vi "fgv - fast counter.vi"(8 "error in (no error)":errorcluster, 10 "Write Data (0)":u16, 11 "Operation":enum16{"Read", "Write"}(ring)) -> (0 "error out":errorcluster, 2 "Read Data":u16)   [LabVIEW 2016]
panel:
  # "fgv - fast counter"
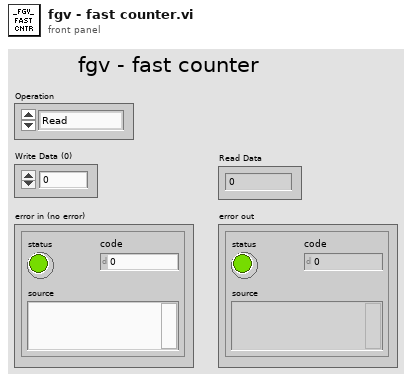
[diagram p1: front panel]
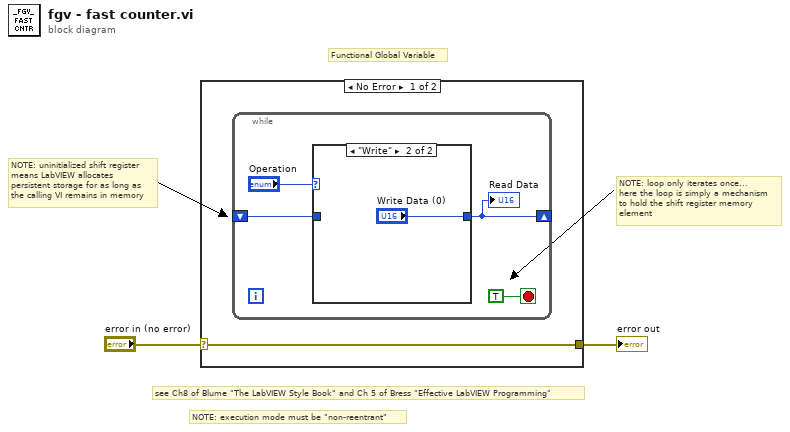
[diagram p0: block diagram]
diagram:
  # "Functional Global Variable"
  # "NOTE: loop only iterates once...\nhere the loop is simply a mechanism\nto hold the shift register memory\nelement"
  # "NOTE: uninitialized shift register\nmeans LabVIEW allocates\npersistent storage for as long as\nthe calling VI remains in memory"
  # "NOTE: execution mode must be \"non-reentrant\""
  # "see Ch8 of Blume \"The LabVIEW Style Book\" and Ch 5 of Bress \"Effective LabVIEW Programming\""
  n1 = case shown="No Error" "error in (no error)" {
    selector: "error in (no error)" -> [w3 w10]
    tunnel: [w3 w10] -> w1
    frame No Error {
      n2 = while {
        shift-right: [w6] -> _
        shift-left: _ -> [w5]
        stop <- TRUE stop-if-true
        n3 = case shown="\"Write\"" "Operation" {
          tunnel: [w8 "Write Data (0)"] -> w6
          tunnel: w5 -> [w8 _]
          frame "Read", Default {
          }
          frame "Write" {
          }
        }
        "Read Data" <- w6
      }
    }
    frame Error {
    }
  }
  "error out" <- w1
